vi "Command to Array.vi"(0 "Input command":string="Write to VISA, \u0000\u0000\u0000\u000eGPIB::12::inst, , offoff") -> (7 "parameter array":string[](array[string]), 8 "Identifield command":string="Write to VISA")   [LabVIEW 2020]
panel:
  # "Note: The VISA address is included parameter array. Library2.vi treats the VISA address separately."
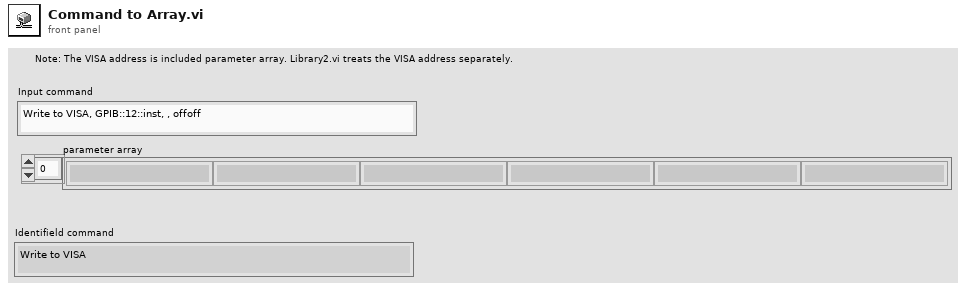
[diagram p1: front panel]
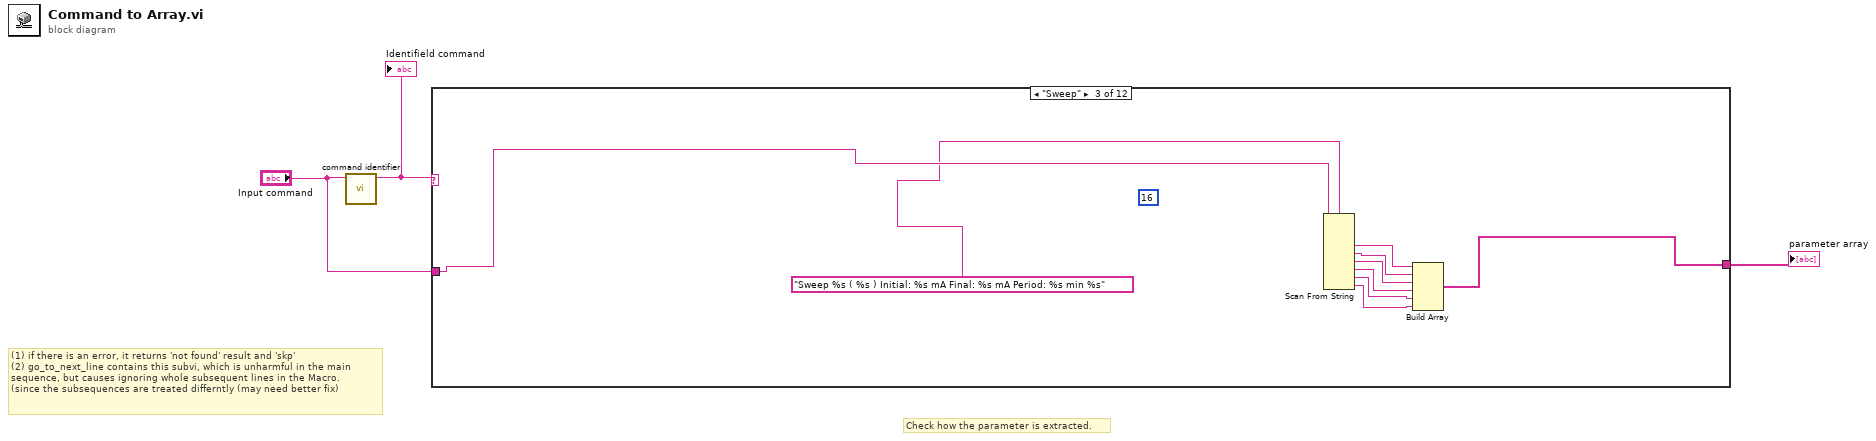
[diagram p0: block diagram]
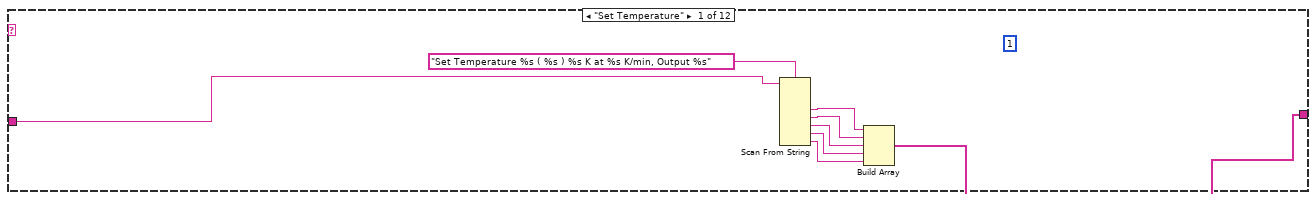
[diagram p2: hidden frame]
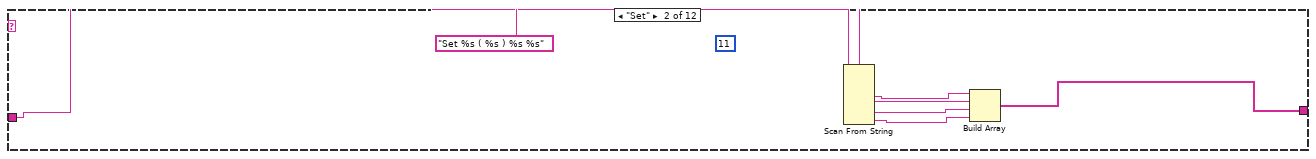
[diagram p3: hidden frame]
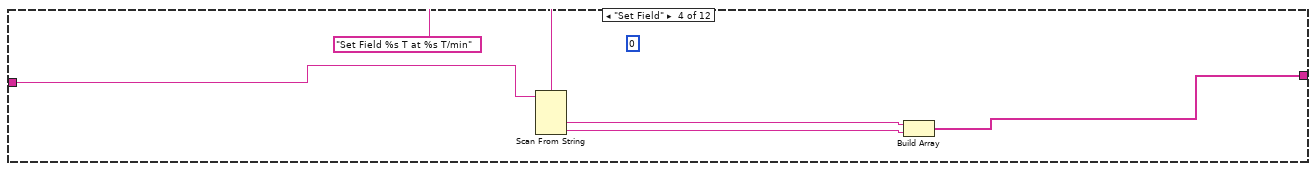
[diagram p4: hidden frame]
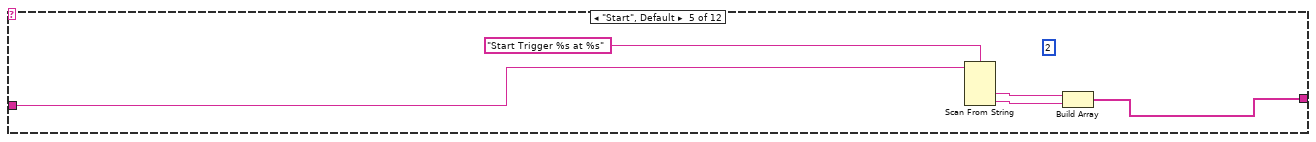
[diagram p5: hidden frame]
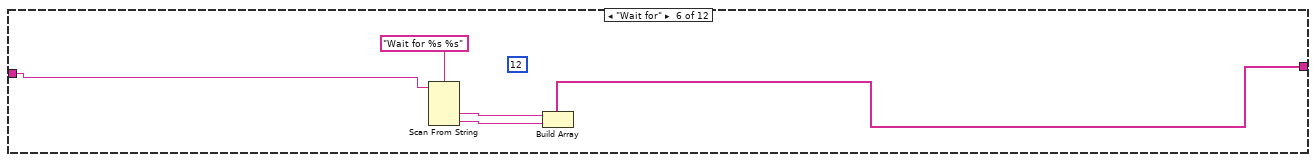
[diagram p6: hidden frame]
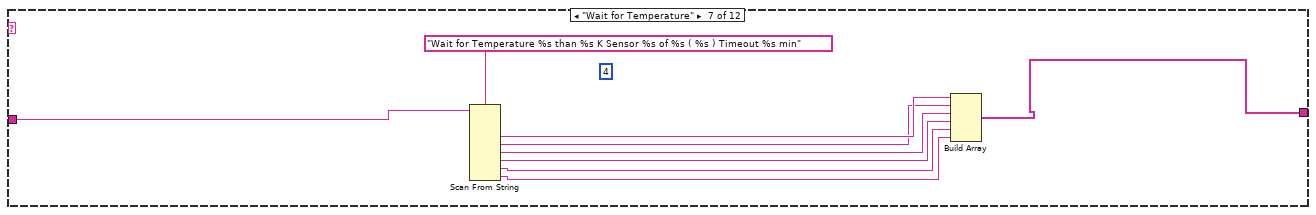
[diagram p7: hidden frame]
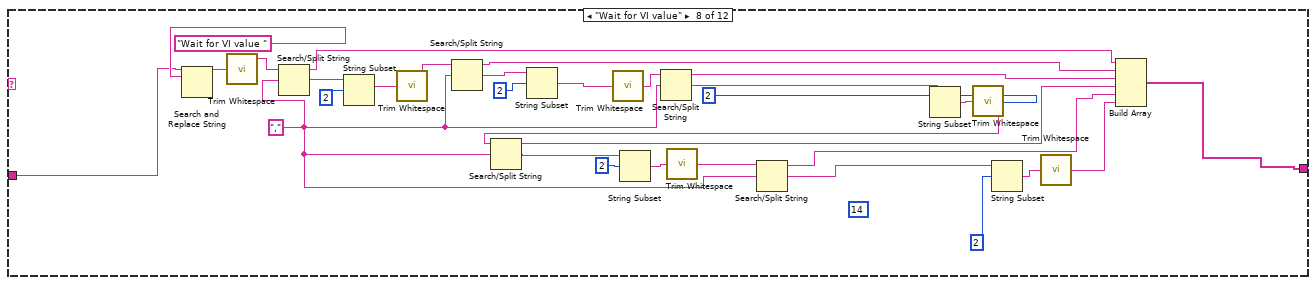
[diagram p8: hidden frame]
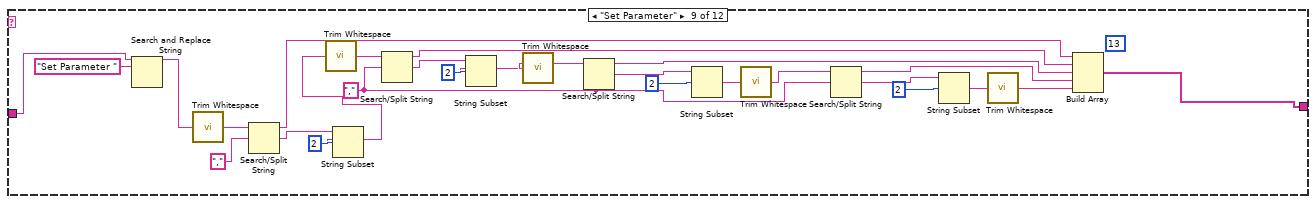
[diagram p9: hidden frame]
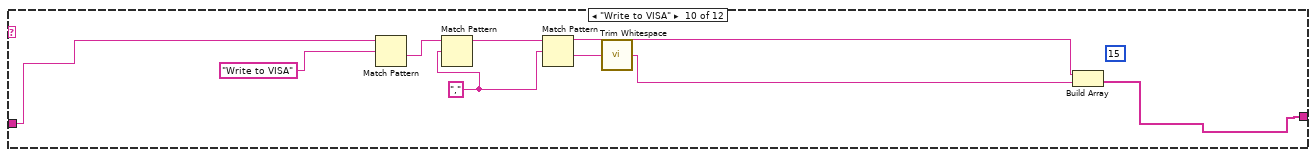
[diagram p10: hidden frame]
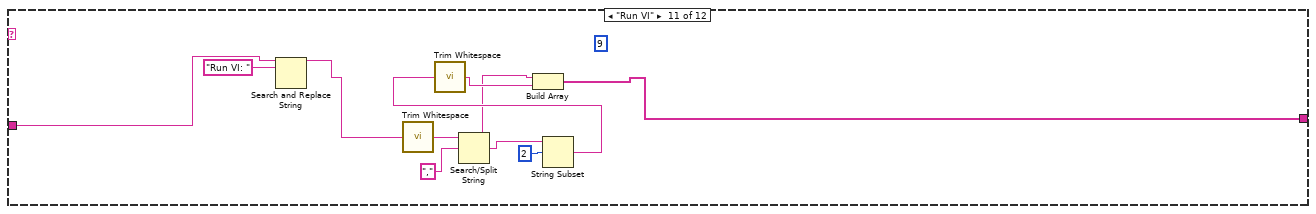
[diagram p11: hidden frame]
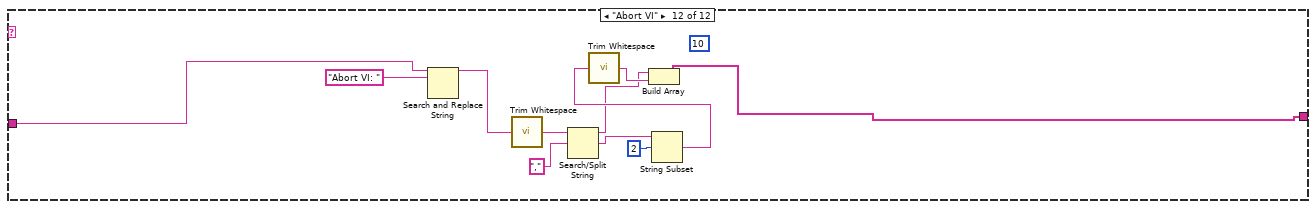
[diagram p12: hidden frame]
diagram:
  # "(1) if there is an error, it returns 'not found' result and 'skp'\n(2) go_to_next_line contains this subvi, which is unharmful in the main\nsequence, but causes ignoring whole subsequent lines in the Macro. \n(since the subsequences are treated differntly (may need better fix)"
  # "Check how the parameter is extracted."
  n1 = call "command identifier.vi"("Input command"="Input command") -> ("Identifield command"=w3:string)  [unwired: 10 in]
  "Identifield command" <- w3
  n2 = case shown="\"Sweep\"" w3 {
    tunnel: "Input command" -> [w7 w15 w25 w29 w34 w39 w46 w60 w91 w113 w128 w139]
    tunnel: [w6 w14 w21 w28 w33 w38 w45 w52 w83 w110 w119 w130] -> w2
    frame "Set Temperature" {
      (unwired) 1 ("No. of command")
      n3 = Scan From String(format string="Set Temperature %s ( %s ) %s K at %s K/min, Output %s", input string=w7) -> (output 1=w5:string, output 2=w4:string, output 3=w10:string, output 4=w9:string, output 5=w8:string)  [unwired: 7 in, 3 out]
      n4 = Build Array(w5, w4, w10, w9, w8) -> (w6:string[])
    }
    frame "Set" {
      (unwired) 11 ("No. of command")
      n5 = Scan From String(format string="Set %s ( %s ) %s %s", input string=w15) -> (output 1=w13:string, output 2=w12:string, output 3=w17:string, output 4=w16:string)  [unwired: 6 in, 3 out]
      n6 = Build Array(w13, w12, w17, w16) -> (w14:string[])
    }
    frame "Sweep" {
      (unwired) 16 ("No. of command")
      n7 = Scan From String(format string="Sweep %s ( %s ) Initial: %s mA Final: %s mA Period: %s min %s", input string=w25) -> (output 1=w20:string, output 2=w19:string, output 3=w27:string, output 4=w26:string, output 5=w24:string, output 6=w23:string)  [unwired: 8 in, 3 out]
      n8 = Build Array(w20, w19, w27, w26, w24, w23) -> (w21:string[])
    }
    frame "Set Field" {
      (unwired) 0 ("No. of command")
      n9 = Scan From String(format string="Set Field %s T at %s T/min", input string=w29) -> (output 1=w31:string, output 2=w30:string)  [unwired: 4 in, 3 out]
      n10 = Build Array(w31, w30) -> (w28:string[])
    }
    frame "Start", Default {
      (unwired) 2 ("No. of command")
      n11 = Scan From String(format string="Start Trigger %s at %s", input string=w34) -> (output 1=w36:string, output 2=w35:string)  [unwired: 4 in, 3 out]
      n12 = Build Array(w36, w35) -> (w33:string[])
    }
    frame "Wait for" {
      (unwired) 12 ("No. of command")
      n13 = Scan From String(format string="Wait for %s %s", input string=w39) -> (output 1=w41:string, output 2=w40:string)  [unwired: 4 in, 3 out]
      n14 = Build Array(w41, w40) -> (w38:string[])
    }
    frame "Wait for Temperature" {
      (unwired) 4 ("No. of command")
      n15 = Scan From String(format string="Wait for Temperature %s than %s K Sensor %s of %s ( %s ) Timeout %s min", input string=w46) -> (output 1=w50:string, output 2=w49:string, output 3=w48:string, output 4=w47:string, output 5=w44:string, output 6=w43:string)  [unwired: 8 in, 3 out]
      n16 = Build Array(w50, w49, w48, w47, w44, w43) -> (w45:string[])
    }
    frame "Wait for VI value" {
      w58 = "," ("search string/char (-)")
      (unwired) 14 ("No. of command")
      n17 = Search and Replace String(input string=w60, search string="Wait for VI value ") -> (result string=w65:string)  [unwired: 6 in, 3 out]
      n18 = call <vilib>:"Trim Whitespace.vi"("string"=w65) -> ("trimmed string"=w59:string)  [unwired: 1 in]
      n19 = Search/Split String(string=w59, search string/char (-)=w58) -> (substring before match=w53:string, match + rest of string=w56:string)  [unwired: 1 in, 1 out]
      n20 = String Subset(string=w56, offset (0)=2) -> (substring=w55:string)  [unwired: 1 in]
      n21 = call <vilib>:"Trim Whitespace.vi"("string"=w55) -> ("trimmed string"=w54:string)  [unwired: 1 in]
      n22 = Search/Split String(string=w54, search string/char (-)=w58) -> (substring before match=w79:string, match + rest of string=w67:string)  [unwired: 1 in, 1 out]
      n23 = String Subset(string=w67, offset (0)=2) -> (substring=w68:string)  [unwired: 1 in]
      n24 = call <vilib>:"Trim Whitespace.vi"("string"=w68) -> ("trimmed string"=w63:string)  [unwired: 1 in]
      n25 = Search/Split String(string=w63, search string/char (-)=w58) -> (substring before match=w80:string, match + rest of string=w70:string)  [unwired: 1 in, 1 out]
      n26 = String Subset(string=w70, offset (0)=2) -> (substring=w71:string)  [unwired: 1 in]
      n27 = call <vilib>:"Trim Whitespace.vi"("string"=w71) -> ("trimmed string"=w64:string)  [unwired: 1 in]
      n28 = Search/Split String(string=w64, search string/char (-)=w58) -> (substring before match=w81:string, match + rest of string=w76:string)  [unwired: 1 in, 1 out]
      n29 = String Subset(string=w76, offset (0)=2) -> (substring=w75:string)  [unwired: 1 in]
      n30 = call <vilib>:"Trim Whitespace.vi"("string"=w75) -> ("trimmed string"=w77:string)  [unwired: 1 in]
      n31 = Search/Split String(string=w77, search string/char (-)=w58) -> (substring before match=w82:string, match + rest of string=w78:string)  [unwired: 1 in, 1 out]
      n32 = String Subset(string=w78, offset (0)=2) -> (substring=w73:string)  [unwired: 1 in]
      n33 = call <vilib>:"Trim Whitespace.vi"("string"=w73) -> ("trimmed string"=w62:string)  [unwired: 1 in]
      n34 = Build Array(w53, w79, w80, w81, w82, w62) -> (w52:string[])
    }
    frame "Set Parameter" {
      w104 = "," ("search string/char (-)")
      (unwired) 13 ("No. of command")
      n35 = Search and Replace String(input string=w91, search string="Set Parameter ") -> (result string=w86:string)  [unwired: 6 in, 3 out]
      n36 = call <vilib>:"Trim Whitespace.vi"("string"=w86) -> ("trimmed string"=w89:string)  [unwired: 1 in]
      n37 = Search/Split String(string=w89, search string/char (-)=",") -> (substring before match=w84:string, match + rest of string=w87:string)  [unwired: 1 in, 1 out]
      n38 = String Subset(string=w87, offset (0)=2) -> (substring=w85:string)  [unwired: 1 in]
      n39 = call <vilib>:"Trim Whitespace.vi"("string"=w85) -> ("trimmed string"=w101:string)  [unwired: 1 in]
      n40 = Search/Split String(string=w101, search string/char (-)=w104) -> (substring before match=w108:string, match + rest of string=w99:string)  [unwired: 1 in, 1 out]
      n41 = String Subset(string=w99, offset (0)=2) -> (substring=w98:string)  [unwired: 1 in]
      n42 = call <vilib>:"Trim Whitespace.vi"("string"=w98) -> ("trimmed string"=w107:string)  [unwired: 1 in]
      n43 = Search/Split String(string=w107, search string/char (-)=w104) -> (substring before match=w106:string, match + rest of string=w96:string)  [unwired: 1 in, 1 out]
      n44 = String Subset(string=w96, offset (0)=2) -> (substring=w95:string)  [unwired: 1 in]
      n45 = call <vilib>:"Trim Whitespace.vi"("string"=w95) -> ("trimmed string"=w105:string)  [unwired: 1 in]
      n46 = Search/Split String(string=w105, search string/char (-)=w104) -> (substring before match=w103:string, match + rest of string=w93:string)  [unwired: 1 in, 1 out]
      n47 = String Subset(string=w93, offset (0)=2) -> (substring=w92:string)  [unwired: 1 in]
      n48 = call <vilib>:"Trim Whitespace.vi"("string"=w92) -> ("trimmed string"=w102:string)  [unwired: 1 in]
      n49 = Build Array(w84, w108, w106, w103, w102) -> (w83:string[])
    }
    frame "Write to VISA" {
      w115 = "," ("search string/char (-)")
      (unwired) 15 ("No. of command")
      n50 = Match Pattern(string=w113, regular expression="Write to VISA" ("search string")) -> (after substring=w116:string)  [unwired: 1 in, 3 out]
      n51 = Match Pattern(string=w116, regular expression=w115) -> (after substring=w117:string)  [unwired: 1 in, 3 out]
      n52 = Match Pattern(string=w117, regular expression=w115) -> (before substring=w112:string, after substring=w118:string)  [unwired: 1 in, 2 out]
      n53 = call <vilib>:"Trim Whitespace.vi"("string"=w118) -> ("trimmed string"=w111:string)  [unwired: 1 in]
      n54 = Build Array(w112, w111) -> (w110:string[])
    }
    frame "Run VI" {
      (unwired) 9 ("No. of command")
      n55 = Search and Replace String(input string=w128, search string="Run VI: ") -> (result string=w123:string)  [unwired: 6 in, 3 out]
      n56 = call <vilib>:"Trim Whitespace.vi"("string"=w123) -> ("trimmed string"=w126:string)  [unwired: 1 in]
      n57 = Search/Split String(string=w126, search string/char (-)=",") -> (substring before match=w120:string, match + rest of string=w124:string)  [unwired: 1 in, 1 out]
      n58 = String Subset(string=w124, offset (0)=2) -> (substring=w122:string)  [unwired: 1 in]
      n59 = call <vilib>:"Trim Whitespace.vi"("string"=w122) -> ("trimmed string"=w121:string)  [unwired: 1 in]
      n60 = Build Array(w120, w121) -> (w119:string[])
    }
    frame "Abort VI" {
      (unwired) 10 ("No. of command")
      n61 = Search and Replace String(input string=w139, search string="Abort VI: " ("format string")) -> (result string=w134:string)  [unwired: 6 in, 3 out]
      n62 = call <vilib>:"Trim Whitespace.vi"("string"=w134) -> ("trimmed string"=w137:string)  [unwired: 1 in]
      n63 = Search/Split String(string=w137, search string/char (-)=",") -> (substring before match=w131:string, match + rest of string=w135:string)  [unwired: 1 in, 1 out]
      n64 = String Subset(string=w135, offset (0)=2) -> (substring=w133:string)  [unwired: 1 in]
      n65 = call <vilib>:"Trim Whitespace.vi"("string"=w133) -> ("trimmed string"=w132:string)  [unwired: 1 in]
      n66 = Build Array(w131, w132) -> (w130:string[])
    }
  }
  "parameter array" <- w2
